vi "Init.vi"(8 "Serial Configuration":T1={"Baud Rate"=9600, "Parity"=0, "Data Bits"=8, "Stop Bits"=10, "Flow Control"=2} {"Flow Control" items=["None", "XON/XOFF", "RTS/CTS", "XON/XOFF & RTS/CTS", "DTR/DSR", "XON/XOFF & DTR/DSR"]; "Stop Bits" items=["1.0"=10, "1.5"=15, "2.0"=20]; "Data Bits" items=["7"=7, "8"=8]; "Parity" items=["None", "Odd", "Even", "Mark", "Space"]; "Baud Rate" items=["300"=300, "600"=600, "1200"=1200, "2400"=2400, "4800"=4800, "9600"=9600, "19200"=19200]}, 9 "General Settings:Timeout Value":u32=10000, 11 "VISA Refnum in":refnum<visa-resource-name>) -> (0 "error out":errorcluster, 1 "serial?":bool, 3 "VISA Refnum out":refnum<visa-resource-name>)   [LabVIEW 2013]
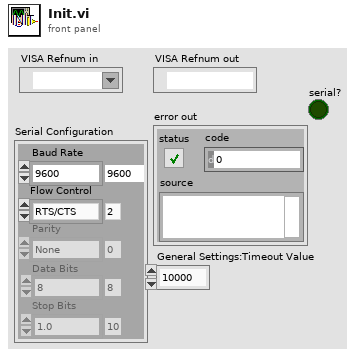
[diagram p1: front panel]
types:
  T1 = cluster{"Baud Rate":u32, "Parity":u16, "Data Bits":u16, "Stop Bits":u16, "Flow Control":u16}
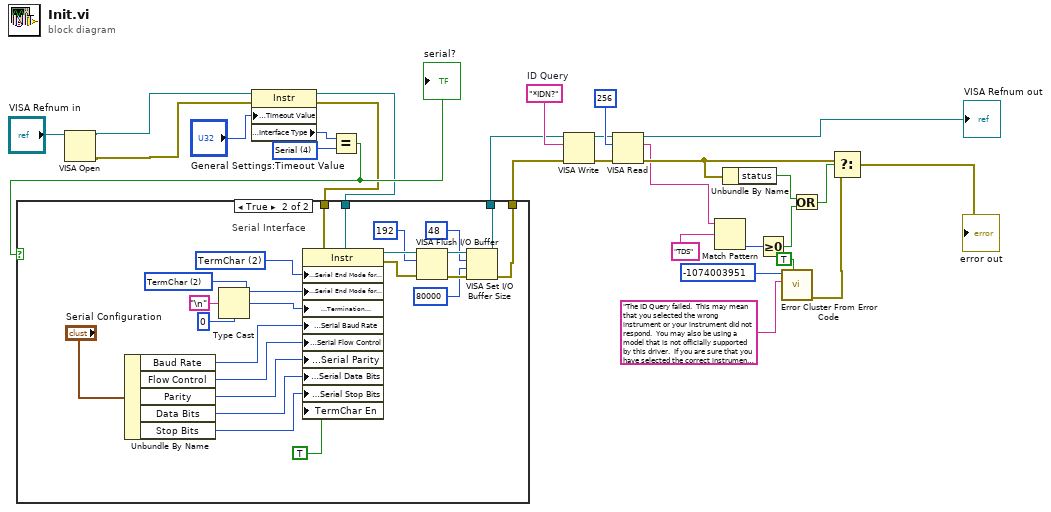
[diagram p0: block diagram]
diagram:
  w11 = u16 4 items=["GPIB"=1, "VXI"=2, "GPIB-VXI"=3, "Serial"=4, "PXI"=5, "TCPIP"=6, "USB"=7] ("Interface Information:Interface Type")
  w18 = "*IDN?"  # ID Query
  n1 = VISA Open(VISA resource name="VISA Refnum in") -> (VISA resource name=w2:refnum<visa-resource-name>, error out=w1:errorcluster)  [unwired: 4 in]
  n2 = property class="Instr"(reference=w2, error in=w1, "General Settings:Timeout Value"="General Settings:Timeout Value") -> (reference out=w8:refnum<visa-resource-name>, error out=w9:errorcluster, "Interface Information:Interface Type"=w12:u16)
  n3 = Equal?(x=w12, y=w11) -> (x = y?=w10:bool)
  "serial?" <- w10
  n4 = case shown="True" w10 {
    tunnel: [w29 w50] -> w7
    tunnel: [w30 w47] -> w6
    tunnel: w8 -> [w29 w52]
    tunnel: w9 -> [w30 w53]
    frame False {
      # "EDIT: Remove interfaces not\nsupported by your instrument."
      # "GPIB, TCP/IP, and USB Interface"
    }
    frame True {
      w31 = u16 2 items=["None", "Last Bit", "TermChar"] ("Serial Settings:End Mode for Reads")
      w40 = u16 2 items=["None", "LastBit", "TermChar"] ("Serial Settings:Serial End Mode for Reads")
      # "Serial Interface"
      n5 = Unbundle By Name("Serial Configuration") -> ("Baud Rate"=w38:u32, "Flow Control"=w34:u16, "Parity"=w36:u16, "Data Bits"=w37:u16, "Stop Bits"=w33:u16)
      n6 = Type Cast(type=u8 0, x="\n" ("Line Feed Constant")) -> (*(type *) &x=w39:u8)
      n7 = property class="Instr"(reference=w52, error in=w53, "Serial Settings:Serial End Mode for Reads"=w31, "Serial Settings:Serial End Mode for Writes"=w40, "Message Based Settings:Termination Character"=w39, "Serial Settings:Serial Baud Rate"=w38, "Serial Settings:Serial Flow Control"=w34, "Serial Settings:Serial Parity"=w36, "Serial Settings:Serial Data Bits"=w37, "Serial Settings:Serial Stop Bits"=w33, "TermChar En"=TRUE ("Message Based Settings:Termination Character Enable")) -> (reference out=w46:refnum<visa-resource-name>, error out=w49:errorcluster)
      n8 = VISA Flush I/O Buffer(VISA resource name=w46, mask (16)=u16 192, error in (no error)=w49) -> (VISA resource name out=w51:refnum<visa-resource-name>, error out=w48:errorcluster)
      n9 = VISA Set I/O Buffer Size(VISA resource name=w51, mask (16)=u16 48, size (4096)=u32 80000 ("size (0)"), error in (no error)=w48) -> (VISA resource name out=w50:refnum<visa-resource-name>, error out=w47:errorcluster)
    }
  }
  n10 = VISA Write(VISA resource name=w7, write buffer=w18, error in (no error)=w6) -> (VISA resource name out=w14:refnum<visa-resource-name>, error out=w15:errorcluster)  [unwired: 1 out]
  n11 = VISA Read(VISA resource name=w14, byte count=u32 256, error in (no error)=w15) -> (VISA resource name out=→"VISA Refnum out":refnum<visa-resource-name>, read buffer=w3:string, error out=w26:errorcluster)  [unwired: 1 out]
  n12 = Match Pattern(string=w3, regular expression="TDS") -> (offset past match=w4:i32)  [unwired: 1 in, 3 out]
  n13 = Unbundle By Name(w26) -> ("status"=w23:bool)
  n14 = Greater Or Equal To 0?(x=w4) -> (x >= 0?=w24:bool)
  n15 = call <vilib>:"Error Cluster From Error Code.vi"("show call chain? (False)"=TRUE, "error message (\"\")"="The ID Query failed.  This may mean that you selected the wrong instrument or your instrument did not respond.  You may also be using a model that is not officially supported by this driver.  If you are sure that you have selected the correct instrument and it is responding, try disabling the ID Query." ("Source (VI Name)"), "error code (0)"=-1074003951 ("Code")) -> ("error out"=w19:errorcluster)  [unwired: 6 in]
  n16 = Or(x=w23, y=w24) -> (x .or. y?=w25:bool)
  n17 = Select(t=w26, s=w25, f=w19) -> (s? t:f=→"error out":errorcluster)
